vi "Rising Edge Detector.vi"(1 "Input":bool) -> (0 "Rising edge?":bool)   [LabVIEW 2015]
doc: "Emits True when input changes from False -> True"
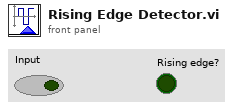
[diagram p1: front panel]
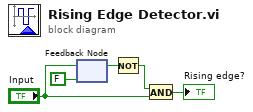
[diagram p0: block diagram]
diagram:
  n1 = feedback-in #1("Input") -> ()
  n2 = feedback #1(FALSE ("Input")) -> (w5:bool)
  n3 = Not(x=w5) -> (.not. x?=w1:bool)
  n4 = And(x=w1, y="Input") -> (x .and. y?=→"Rising edge?":bool)
